vi "CTRE_PigeonIMU_GetTempStateUpTime.vi"(8 "error in (no error)":errorcluster, 11 "PigeonIMUDevRef":T4={"DeviceStatus"={"status"=FALSE, "code"=0, "source"=""}, "Device Number"=0, "Type"=352321536, "Device ID"=0, "Handle"=0, "UsageFrame"=0, "Library Path"=path ""} {"Type" items=["CAN"=352321536, "TalonSRX"=33554432]}) -> (0 "error out":errorcluster, 2 "Temp/State/UpTime":T3 {"CurrentMode" items=["BootTareGryoAccel"=0, "Temperature"=1, "Magnetometer12Pt"=2, "Magnetometer360"=3, "Accelerometer"=5]}, 3 "PigeonIMUDevRef":T4={"DeviceStatus"={"status"=FALSE, "code"=0, "source"=""}, "Device Number"=0, "Type"=352321536, "Device ID"=0, "Handle"=0, "UsageFrame"=0, "Library Path"=path ""} {"Type" items=["CAN"=352321536, "TalonSRX"=33554432]})   [LabVIEW 2016]
uses:
  CTRE_PigeonIMU_CalibrationMode.ctl
  CTRE_PigeonIMU_DeviceRef.ctl
  CTRE_PigeonIMU_ConnectionType.ctl
  CTRE_PigeonIMU_PigeonState.ctl
  CTRE_PigeonIMU_MessageIDs.ctl
panel:
  in  "CalibrationMode":T1 items=["BootTareGryoAccel"=0, "Temperature"=1, "Magnetometer12Pt"=2, "Magnetometer360"=3, "Accelerometer"=5]
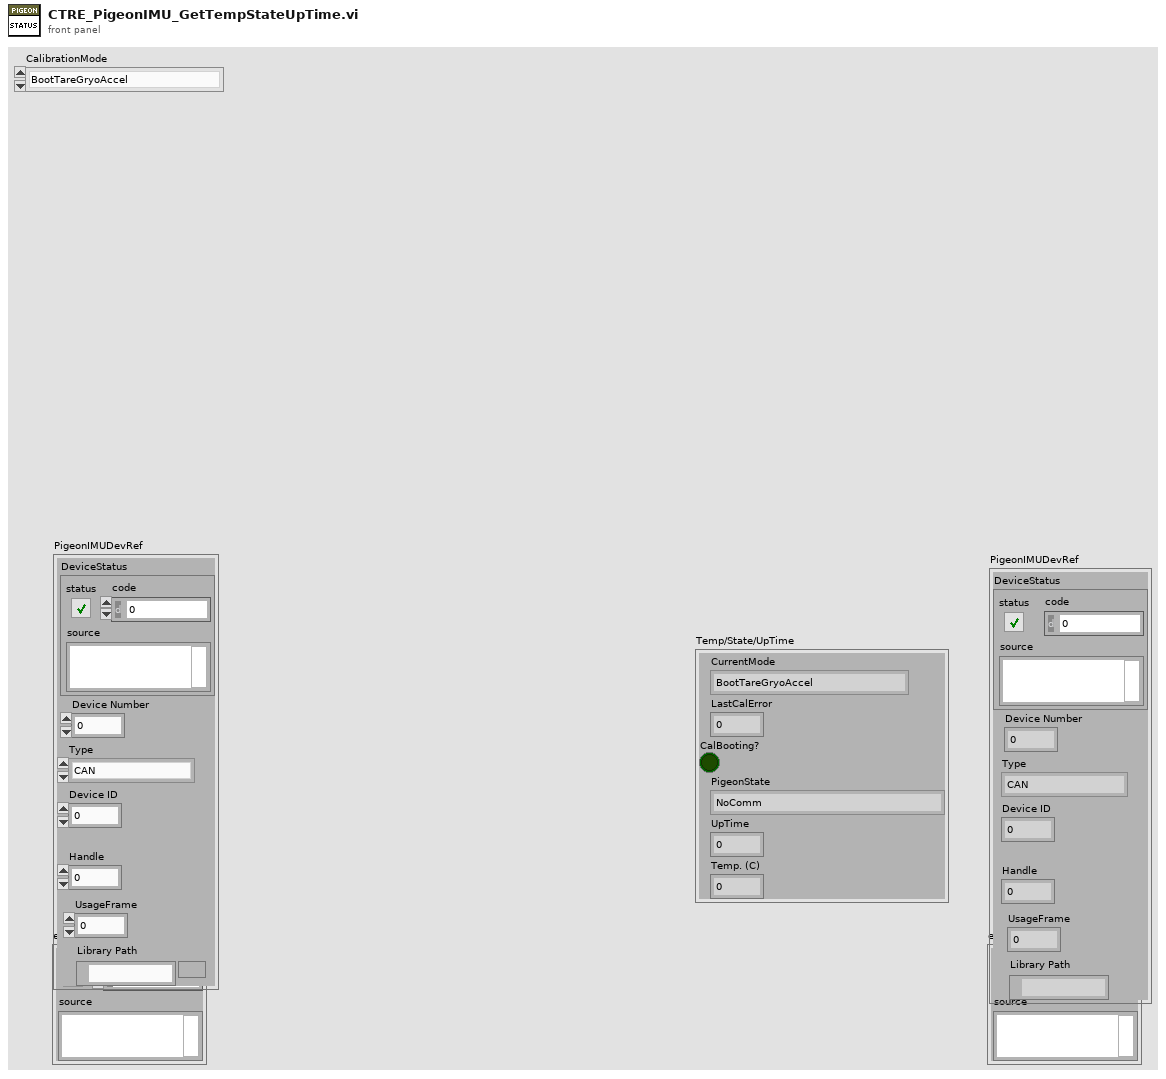
[diagram p1: front panel]
types:
  T1 = typedef "CTRE_PigeonIMU_CalibrationMode.ctl" = u16
  T2 = typedef "CTRE_PigeonIMU_PigeonState.ctl" = enum16{"NoComm", "Initializing", "Ready", "UserCalibration"}
  T3 = cluster{"CurrentMode":T1, "LastCalError":i32, "CalBooting?":bool, "PigeonState":T2, "UpTime":u32, "Temp. (C)":dbl}
  T4 = typedef "CTRE_PigeonIMU_DeviceRef.ctl" = cluster{"DeviceStatus":errorcluster, "Device Number":u8, "Type":T5, "Device ID":u32, "Handle":u64, "UsageFrame":u32, "Library Path":path}
  T5 = typedef "CTRE_PigeonIMU_ConnectionType.ctl" = u32
  T6 = typedef "CTRE_PigeonIMU_MessageIDs.ctl" = u32
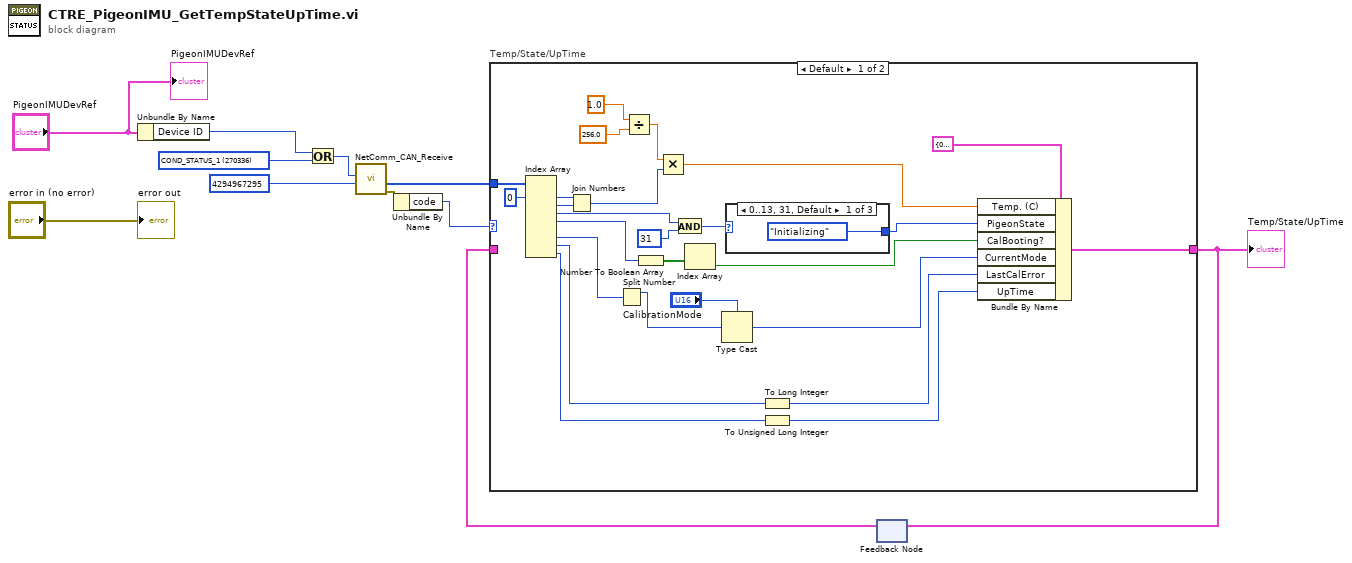
[diagram p0: block diagram]
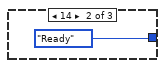
[diagram p2: hidden frame]
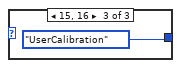
[diagram p3: hidden frame]
diagram:
  w9 = T6 270336 items=["RAW_STATUS_2"=265280, "RAW_STATUS_4"=265408, "RAW_STATUS_6"=265536, "BIASED_STATUS_2"=269376, "BIASED_STATUS_4"=269504, "BIASED_STATUS_6"=269632, "COND_STATUS_1"=270336, "COND_STATUS_2"=270400, "COND_STATUS_3"=270464, "COND_STATUS_4"=270528, "COND_STATUS_5"=270592, "COND_STATUS_6"=270656, "COND_STATUS_7"=270720, "COND_STATUS_8"=270784, "COND_STATUS_9"=270848, "COND_STATUS_10"=270912, "CONTROL_1"=272384, "PARAM_REQUEST"=273408, "PARAM_RESPONSE"=273472, "PARAM_SET"=273536] ("MessageIDs")
  n1 = Unbundle By Name("PigeonIMUDevRef") -> ("Device ID"=w5:u32)
  n2 = Or(x=w5, y=w9) -> (x .or. y?=w8:T6)
  n3 = call <vilib>:"NetComm_CAN_Receive.vi"("Message ID Mask"=u32 4294967295, "Message ID"=w8) -> ("error out"=w2:errorcluster, "Data"=w10:u8[])  [unwired: 6 in, 2 out]
  n4 = Unbundle By Name(w2) -> ("code"=w1:i32)
  n5 = feedback #1() -> (w3:T3)  [unwired: 1 in]
  n6 = case "Temp/State/UpTime" shown="Default" w1 {
    tunnel: w10 -> [w37 _]
    tunnel: [w12 w41] -> w4
    tunnel: w3 -> [_ w41]
    frame Default {
      n7 = Index Array(array=w37, index #1=0 ("index")) -> (element #1=w36:u8, element #2=w35:u8, element #3=w34:u8, element #4=w20:u8, element #6=w17:u8, element #7=w22:u8, element #8=w23:u8)  [unwired: 7 in, 1 out]
      n8 = Join Numbers(hi=w36, lo=w35) -> ((hi.lo)=w28:u16)
      n9 = Split Number(x=w17) -> (hi(x)=w16:u8)  [unwired: 1 out]
      n10 = Divide(x=1.0, y=256.0) -> (x/y=w29:dbl)
      n11 = Number To Boolean Array(number=w20) -> (Boolean array=w19:bool[])
      n12 = Multiply(x=w29, y=w28) -> (x*y=w27:dbl)
      n13 = And(x=w34, y=u8 31) -> (x .and. y?=w33:u8)
      n14 = Index Array(array=w19) -> (element=w18:bool)  [unwired: 1 in]
      n15 = Type Cast(type="CalibrationMode", x=w16) -> (*(type *) &x=w14:T1)
      n16 = case shown="0..13, 31, Default" w33 {
        tunnel: [CTRE_PigeonIMU_PigeonState."Initializing" ("PigeonState") CTRE_PigeonIMU_PigeonState."Ready" ("PigeonState") CTRE_PigeonIMU_PigeonState."UserCalibration" ("PigeonState")] -> w32
        frame 0..13, 31, Default {
        }
        frame 14 {
        }
        frame 15, 16 {
        }
      }
      n17 = To Long Integer(number=w22) -> (32bit integer=w24:i32)
      n18 = To Unsigned Long Integer(number=w23) -> (unsigned 32bit integer=w25:u32)
      n19 = Bundle By Name(cluster=T3 {"CurrentMode"=0, "LastCalError"=0, "CalBooting?"=FALSE, "PigeonState"=enum."NoComm", "UpTime"=0, "Temp. (C)"=0.0} ("Calibration"), "Temp. (C)"=w27, "PigeonState"=w32, "CalBooting?"=w18, "CurrentMode"=w14, "LastCalError"=w24, "UpTime"=w25) -> (w12:T3)
    }
    frame -44087 {
    }
  }
  "Temp/State/UpTime" <- w4
  n20 = feedback-in #1(w4) -> ()
  "PigeonIMUDevRef" <- "PigeonIMUDevRef"
  "error out" <- "error in (no error)"
